vi "user32.getWindowSize.vi"(8 "error in":errorcluster caption="error in (no error)", 9 "hWnd":u32) -> (0 "error out":errorcluster, 1 "hWnd out":u32, 4 "Rectangle Coordinates":T1)   [LabVIEW 2018]
uses:
  User32.dll
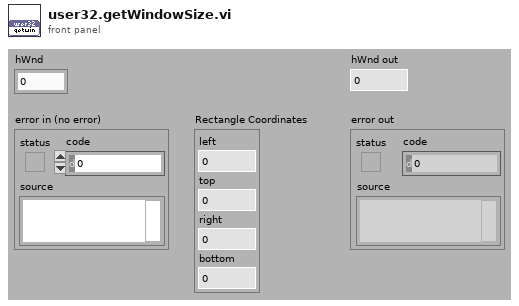
[diagram p1: front panel]
types:
  T1 = cluster{"left":i32, "top":i32, "right":i32, "bottom":i32}
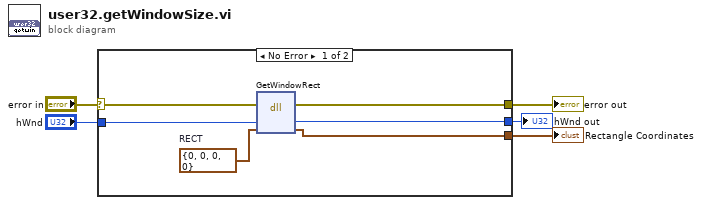
[diagram p0: block diagram]
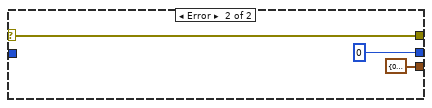
[diagram p2: hidden frame]
diagram:
  n1 = case shown="No Error" "error in" {
    selector: "error in" -> [w9 w14]
    tunnel: [w10 w14] -> w5
    tunnel: "hWnd" -> [w8 _]
    tunnel: [w7 T1 {"left"=0, "top"=0, "right"=0, "bottom"=0} ("IpRect")] -> w2
    tunnel: [w6 0] -> w1
    frame No Error {
      w11 = T1 {"left"=0, "top"=0, "right"=0, "bottom"=0}  # RECT
      n2 = dll-call lib="USER32.DLL" fn="GetWindowRect"(error in=w9, "hWnd"=w8, "IpRect"=w11) -> (error out=w10:errorcluster, "hWnd"=w6:u32, "IpRect"=w7:T1)  [unwired: 3 in, 1 out]
    }
    frame Error {
    }
  }
  "error out" <- w5
  "Rectangle Coordinates" <- w2
  "hWnd out" <- w1
